vi "Deserialize Connections in Wrapper - Multiple Converter.vi"(11 "error in":errorcluster) -> (15 "error out":errorcluster)   [LabVIEW 2021, in "Converter.lvlib"]
uses:
  Converter.lvlib
  <vilib>/Utility/traverseref.llb/TRef TravTarget.ctl
  <vilib>/Utility/miscctls.llb/LVPointTypeDef.ctl
  <vilib>/Utility/traverseref.llb/VI Scripting - Traverse.lvlib
  Converter Reusables/Converter Reusables.lvlib
  Path Functions/Path Functions.lvlib
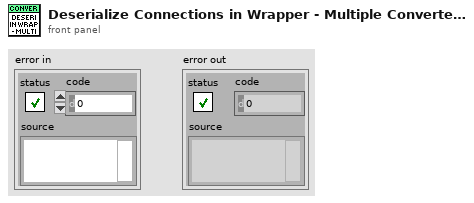
[diagram p1: front panel]
types:
  T1 = typedef "TRef TravTarget.ctl" = enum16{"FP", "BD", "Other"}
  T2 = typedef "LVPointTypeDef.ctl" = cluster{"Horizontal":i16, "Vertical":i16}
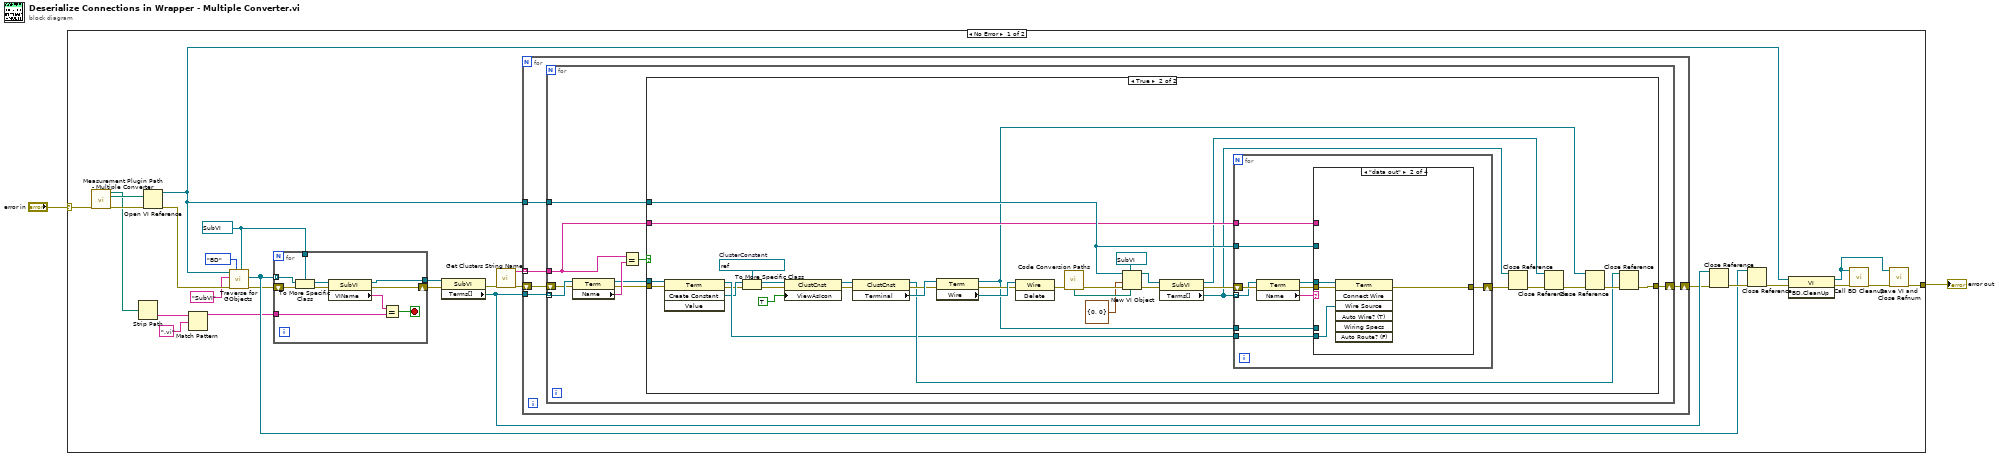
[diagram p0: block diagram]
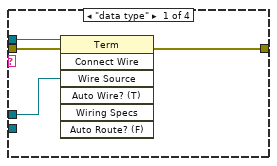
[diagram p3: hidden frame]
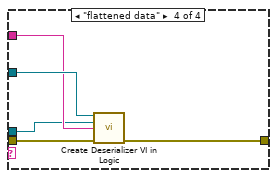
[diagram p5: hidden frame]
diagram:
  n1 = case shown="No Error" "error in" {
    selector: "error in" -> [w29 w113]
    tunnel: [w17 w113] -> w2
    frame No Error {
      w9 = refnum<vi> refnum ("Other Refnum")
      n2 = call "Measurement Plugin Path - Multiple Converter.vi"("error in"=w29) -> ("new code module"=w8:path, "wrapper path"=w28:path, "error out"=w27:errorcluster)  [unwired: 2 in, 10 out]
      n3 = Strip Path(path=w8) -> (name=w7:string)  [unwired: 1 out]
      n4 = Open VI Reference(vi path=w28, error in (no error)=w27) -> (vi reference=w16:refnum<vi>, error out=w26:errorcluster)  [unwired: 4 in]
      n5 = Match Pattern(string=w7, regular expression=".vi") -> (before substring=w5:string)  [unwired: 1 in, 3 out]
      n6 = call <vilib>:"Traverse for GObjects.vi"("Other Refnum"=w9, "Traverse Target"=TRef_TravTarget."BD", "error in (no error)"=w26, "Class Name"="SubVI", "VI Refnum"=w16) -> ("error out"=w10:errorcluster, "References"=w11:refnum<vi>[])  [unwired: 3 in, 2 out]
      n7 = for {
        tunnel: w11 -> [w111] mode=indexing
        tunnel: w9 -> [w110]
        tunnel: w5 -> [w105]
        shift-right: [w104] -> w4
        shift-left: w10 -> [w112]
        tunnel: [w103] -> w3
        stop <- w106 stop-if-true
        n8 = To More Specific Class(target class=w110, reference=w111, error in=w112) -> (specific class reference=w109:refnum<vi>, error out=w108:errorcluster)
        n9 = property class="SubVI"(reference=w109, error in=w108) -> (reference out=w103:refnum<vi>, error out=w104:errorcluster, "VIName"=w107:string)
        n10 = Equal?(x=w107, y=w105) -> (x = y?=w106:bool)
      }
      n11 = property class="SubVI"(reference=w3, error in=w4) -> (error out=w23:errorcluster, "Terms[]"=w20:refnum<vi>[])  [unwired: 1 out]
      n12 = call "Get Clusters String Name.vi"("error in"=w23) -> ("control names out"=w22:string[], "error out"=w21:errorcluster)  [unwired: 12 in, 1 out]
      n13 = for {
        tunnel: w20 -> [w34]
        tunnel: w22 -> [w32] mode=indexing
        shift-right: [w30] -> w19
        shift-left: w21 -> [w33]
        tunnel: w16 -> [w31]
        n14 = for {
          tunnel: w34 -> [w43] mode=indexing
          shift-right: [w36] -> w30
          shift-left: w33 -> [w41]
          tunnel: w32 -> [w35]
          tunnel: w31 -> [w37]
          n15 = property class="Term"(reference=w43, error in=w41) -> (reference out=w38:refnum<vi>, error out=w39:errorcluster, "Name"=w42:string)
          n16 = Equal?(x=w35, y=w42) -> (x = y?=w40:bool)
          n17 = case shown="True" w40 {
            tunnel: w39 -> [w44 w77]
            tunnel: w38 -> [_ w78]
            tunnel: w37 -> [_ w64]
            tunnel: [w44 w55] -> w36
            tunnel: w35 -> [_ w63]
            frame False {
            }
            frame True {
              w50 = refnum<vi> refnum  # ClusterConstant
              n18 = invoke class="Term" method="Create Constant"(reference=w78, error in=w77) -> (reference out=w54:refnum<vi>, error out=w48:errorcluster, "Create Constant"=w52:refnum<vi>)  [unwired: 2 in, 1 out]
              n19 = To More Specific Class(target class=w50, reference=w52, error in=w48) -> (specific class reference=w51:refnum<vi>, error out=w47:errorcluster)
              n20 = property class="ClustCnst"(reference=w51, error in=w47, "ViewAsIcon"=TRUE ("View As Icon")) -> (reference out=w46:refnum<vi>, error out=w45:errorcluster)
              n21 = property class="ClustCnst"(reference=w46, error in=w45) -> (reference out=w56:refnum<vi>, error out=w66:errorcluster, "Terminal"=w68:refnum<vi>)
              n22 = property class="Term"(reference=w68, error in=w66) -> (reference out=w53:refnum<vi>, error out=w65:errorcluster, "Wire"=w67:refnum<vi>)
              n23 = invoke class="Wire" method="Delete"(reference=w67, error in=w65) -> (error out=w76:errorcluster)  [unwired: 1 in, 2 out]
              n24 = call "Code Conversion Paths.vi"("error in"=w76) -> ("deserializer"=w75:path, "error out"=w74:errorcluster)  [unwired: 6 in, 7 out]
              n25 = New VI Object(vi object class=refnum<vi> refnum ("Other Refnum"), owner refnum=w64, position/next to=T2 {"Horizontal"=0, "Vertical"=0} ("location"), 6:w75, 8:w74) -> (object refnum=w71:refnum<vi>, 0:w70:errorcluster)  [unwired: 3 in]
              n26 = property class="SubVI"(reference=w71, error in=w70) -> (reference out=w59:refnum<vi>, error out=w69:errorcluster, "Terms[]"=w61:refnum<vi>[])
              n27 = for {
                tunnel: w61 -> [w85] mode=indexing
                shift-right: [w83] -> w62
                shift-left: w69 -> [w88]
                tunnel: w64 -> [w82]
                tunnel: w63 -> [w81]
                tunnel: w54 -> [w80]
                tunnel: w53 -> [w79]
                n28 = property class="Term"(reference=w85, error in=w88) -> (reference out=w84:refnum<vi>, error out=w87:errorcluster, "Name"=w86:string)
                n29 = case shown="\"data out\"" w86 {
                  tunnel: w87 -> [w91 w96 w97 w102]
                  tunnel: w84 -> [w92 w95 _ w99]
                  tunnel: [w90 w94 w97 w98] -> w83
                  tunnel: w82 -> [_ _ _ w101]
                  tunnel: w81 -> [_ _ _ w100]
                  tunnel: w80 -> [_ w93 _ _]
                  tunnel: w79 -> [w89 _ _ _]
                  frame "data type" {
                    n30 = invoke class="Term" method="Connect Wire"(reference=w92, error in=w91, "Wire Source"=w89) -> (error out=w90:errorcluster)  [unwired: 4 in, 6 out]
                  }
                  frame "data out" {
                    n31 = invoke class="Term" method="Connect Wire"(reference=w95, error in=w96, "Wire Source"=w93) -> (error out=w94:errorcluster)  [unwired: 4 in, 6 out]
                  }
                  frame Default {
                  }
                  frame "flattened data" {
                    n32 = call "Create Deserializer VI in Logic.vi"("vi refnum"=w101, "term refnum"=w99, "name"=w100, "error in"=w102) -> ("error out"=w98:errorcluster)  [unwired: 11 in]
                  }
                }
              }
              n33 = Close Reference(reference=w61, error in (no error)=w62) -> (error out=w60:errorcluster)
              n34 = Close Reference(reference=w59, error in (no error)=w60) -> (error out=w58:errorcluster)
              n35 = Close Reference(reference=w53, error in (no error)=w58) -> (error out=w57:errorcluster)
              n36 = Close Reference(reference=w56, error in (no error)=w57) -> (error out=w55:errorcluster)
            }
          }
        }
      }
      n37 = Close Reference(reference=w20, error in (no error)=w19) -> (error out=w18:errorcluster)
      n38 = Close Reference(reference=w11, error in (no error)=w18) -> (error out=w15:errorcluster)
      n39 = invoke class="VI" method="BD.CleanUp"(reference=w16, error in=w15) -> (reference out=w12:refnum<vi>, error out=w14:errorcluster)  [unwired: 1 in, 1 out]
      n40 = call "Call BD Cleanup.vi"("vi"=w12, "error in"=w14) -> ("error out"=w13:errorcluster)  [unwired: 13 in]
      n41 = call "Save VI and Close Refnum.vi"("vi refnum"=w12, "error in"=w13) -> ("error out"=w17:errorcluster)  [unwired: 13 in]
    }
    frame Error {
    }
  }
  "error out" <- w2
